vi "固定站CODMn测量流程.vi"(11 "控制命令":T1(ring)) -> ()   [LabVIEW 2016, in "斯坦道CODMn.lvlib"]
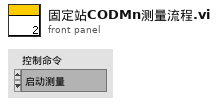
[diagram p1: front panel]
types:
  T1 = enum16{"启动测量", "标样核查", "零点核查", "跨度核查", "空白测试", "平行样测试", "加标回收", "空白校准", "标样校准", "初始化（清洗）", "停止测试", "仪器重启", "校时", "模式设置", "测量间隔设置"}
  T2 = cluster{"仪器":enum16{"", "氨氮", "总磷", "总氮", "CODMn", "CODCr"}, "启动命令":enum16{"启动水样流程", "启动加标流程", "排液", "停止", "柱塞泵启动"}}
  T3 = cluster{"时间标识":timestamp, "参数":string, "日志信息":string, "流程参数":string}
  T4 = cluster{"测量模式":enum16{"水样测量", "标样核查", "零点核查", "跨度核查", "空白测试", "加标回收", "平行样", "校零", "校标"}}
  T5 = cluster{"时间标识":timestamp, "设备":string, "日志信息":string, "流程参数":string}
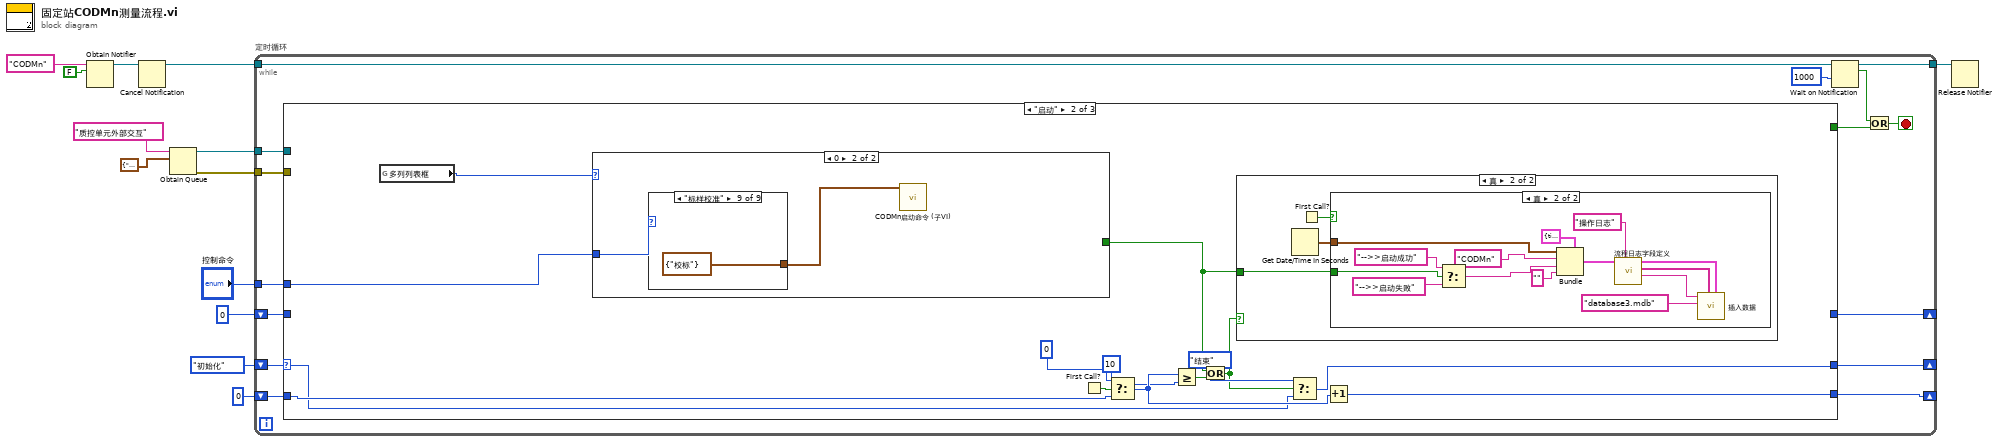
[diagram p0: block diagram]
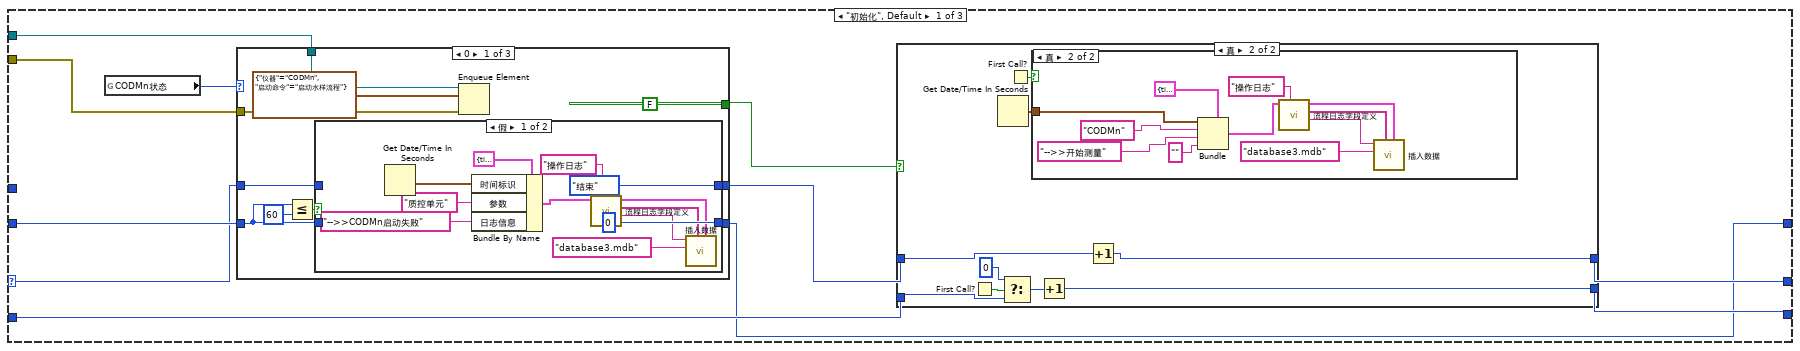
[diagram p2: hidden frame]
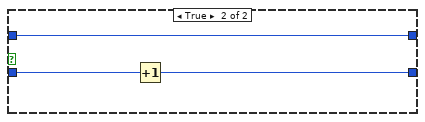
[diagram p5: hidden frame]
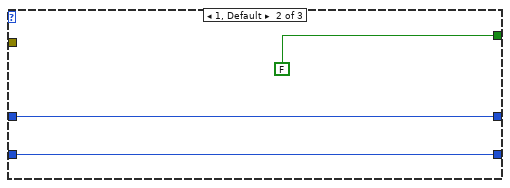
[diagram p6: hidden frame]
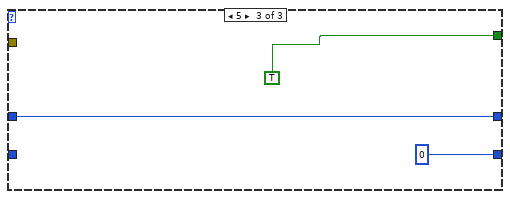
[diagram p7: hidden frame]
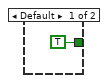
[diagram p10: hidden frame]
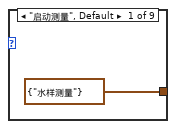
[diagram p11: hidden frame]
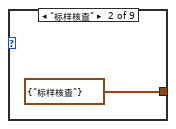
[diagram p12: hidden frame]
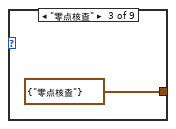
[diagram p13: hidden frame]
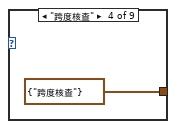
[diagram p14: hidden frame]
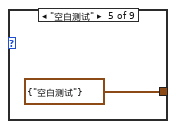
[diagram p15: hidden frame]
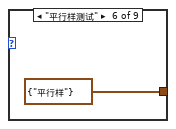
[diagram p16: hidden frame]
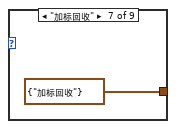
[diagram p17: hidden frame]
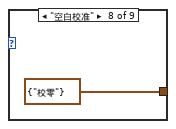
[diagram p18: hidden frame]
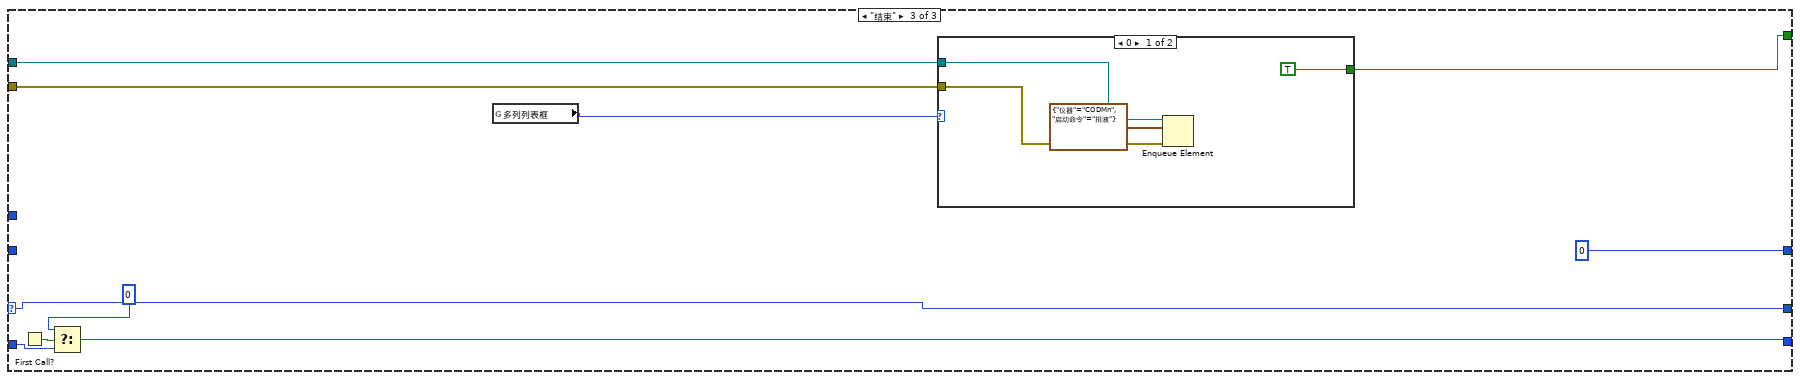
[diagram p19: hidden frame]
diagram:
  n1 = Obtain Notifier(name (unnamed)="CODMn" ("名称（未命名）"), notification data type=FALSE) -> (notifier out=w11:refnum<notifier>)  [unwired: 2 in, 2 out]
  n2 = Cancel Notification(0:w11) -> (8:w10:refnum<notifier>)  [unwired: 1 in, 2 out]
  n3 = Obtain Queue(name (unnamed)="质控单元外部交互" ("名称（未命名）"), element data type=T2 {"仪器"=enum."氨氮", "启动命令"=enum."启动水样流程"} ("元素")) -> (queue out=w3:refnum<queue>, error out=w2:errorcluster)  [unwired: 3 in, 1 out]
  n4 = while "定时循环" {
    tunnel: w10 -> [w28]
    tunnel: "控制命令" -> [w23]
    shift-right: [w22] -> _
    shift-left: enum16{"初始化", "启动", "结束"}."初始化" -> [w24]
    shift-right: [w20] -> _
    shift-left: 0 -> [w21]
    tunnel: [w18] -> w7
    tunnel: w3 -> [w17]
    tunnel: w2 -> [w16]
    shift-right: [w14] -> _
    shift-left: 0 -> [w15]
    stop <- w25 stop-if-true
    n5 = case shown="\"启动\"" w24 {
      selector: w24 -> [w31 w98 w145]
      tunnel: w23 -> [_ w106 _]
      tunnel: [w39 w99 w145] -> w22
      tunnel: w21 -> [w38 w103 w142]
      tunnel: [w37 w102 w141] -> w20
      tunnel: [_ _ w138] -> w19
      tunnel: w17 -> [w35 _ w140]
      tunnel: w16 -> [w34 _ w139]
      tunnel: w15 -> [w33 _ _]
      tunnel: [w32 _ 0] -> w14
      frame "初始化", Default {
        n6 = global read "CODMN外部API.vi" "CODMn状态"() -> (w29:u16)
        n7 = case shown="0" w29 {
          tunnel: [FALSE ("s") FALSE ("s") TRUE ("s")] -> w36
          tunnel: w35 -> [w70 _ _]
          tunnel: w34 -> [w69 _ _]
          tunnel: w33 -> [w67 w87 _]
          tunnel: [w64 w87 0] -> w32
          tunnel: w31 -> [w63 w88 w91]
          tunnel: [w62 w88 w91] -> w30
          frame 0 {
            n8 = Less Or Equal?(x=w67, y=60) -> (x <= y?=w65:bool)
            n9 = case shown="假" w65 {
              tunnel: w67 -> [_ w86]
              tunnel: [0 w85] -> w64
              tunnel: w63 -> [_ w84]
              tunnel: [enum16{"初始化", "启动", "结束"}."结束" w84] -> w62
              frame False {
                n10 = Get Date/Time In Seconds() -> (seconds since 1Jan1904=w79:timestamp)
                n11 = Bundle By Name(cluster=T3 {"时间标识"=timestamp(0 s since 1904-01-01), "参数"="", "日志信息"="", "流程参数"=""} ("data in"), "时间标识"=w79, "参数"="质控单元" ("设备"), "日志信息"="-->>CODMn启动失败") -> (w73:T3)
                n12 = call "流程日志字段定义.vi"("table输入"="操作日志", "data in"=w73) -> ("table输出"=w76:string, "columns"=w77:string[], "data out"=w78:T5)  [unwired: 7 in]
                n13 = call "插入数据.vi"("data"=w78, "columns"=w77, "database"="database3.mdb", "table"=w76) -> ()  [unwired: 7 in, 1 out]
              }
              frame True {
                n14 = Increment(x=w86) -> (x+1=w85:i32)
              }
            }
            n15 = Enqueue Element(queue=w70, element=T2 {"仪器"=enum."CODMn", "启动命令"=enum."启动水样流程"} ("元素"), error in (no error)=w69) -> ()  [unwired: 1 in, 3 out]
          }
          frame 1, Default {
          }
          frame 5 {
          }
        }
        n16 = case shown="真" w36 {
          tunnel: w30 -> [w41 w48]
          tunnel: [w41 w47] -> w39
          tunnel: w38 -> [w40 w45]
          tunnel: [w40 w42] -> w37
          frame False {
          }
          frame True {
            n17 = First Call?() -> (First Call?: T/F=w46:bool)
            n18 = Get Date/Time In Seconds() -> (seconds since 1Jan1904=w50:timestamp)
            n19 = Select(t=0, s=w46, f=w45) -> (s? t:f=w43:i32)
            n20 = First Call?() -> (First Call?: T/F=w49:bool)
            n21 = case shown="真" w49 {
              tunnel: w50 -> [_ w58]
              frame False {
              }
              frame True {
                n22 = Bundle(cluster=T3 {"时间标识"=timestamp(0 s since 1904-01-01), "参数"="", "日志信息"="", "流程参数"=""} ("data in"), "时间标识"=w58, "参数"="CODMn" ("设备"), "日志信息"="-->>开始测量", "流程参数"="" ("table输入")) -> (w51:T3)
                n23 = call "流程日志字段定义.vi"("table输入"="操作日志", "data in"=w51) -> ("table输出"=w54:string, "columns"=w53:string[], "data out"=w52:T5)  [unwired: 7 in]
                n24 = call "插入数据.vi"("data"=w52, "columns"=w53, "database"="database3.mdb", "table"=w54) -> ()  [unwired: 7 in, 1 out]
              }
            }
            n25 = Increment(x=w43) -> (x+1=w42:i32)
            n26 = Increment(x=w48) -> (x+1=w47:enum16{"初始化", "启动", "结束"})
          }
        }
      }
      frame "启动" {
        n27 = global read "运行时序全局变量.vi" "多列列表框"() -> (w93:i32)
        n28 = case shown="0" w93 {
          tunnel: w106 -> [_ w126]
          tunnel: [TRUE _] -> w94
          frame Default {
          }
          frame 0 {
            n29 = case shown="\"标样校准\"" w126 {
              tunnel: [T4 {"测量模式"=enum."水样测量"} ("启动测量模式") T4 {"测量模式"=enum."标样核查"} ("启动测量模式") T4 {"测量模式"=enum."零点核查"} ("启动测量模式") T4 {"测量模式"=enum."跨度核查"} ("启动测量模式") T4 {"测量模式"=enum."空白测试"} ("启动测量模式") T4 {"测量模式"=enum."平行样"} ("启动测量模式") T4 {"测量模式"=enum."加标回收"} ("启动测量模式") T4 {"测量模式"=enum."校零"} ("启动测量模式") T4 {"测量模式"=enum."校标"} ("启动测量模式")] -> w125
              frame "启动测量", Default {
              }
              frame "标样核查" {
              }
              frame "零点核查" {
              }
              frame "跨度核查" {
              }
              frame "空白测试" {
              }
              frame "平行样测试" {
              }
              frame "加标回收" {
              }
              frame "空白校准" {
              }
              frame "标样校准" {
              }
            }
            n30 = call "CODMn启动命令 (子VI).vi"("启动测量模式"=w125) -> ()  [unwired: 11 in]
          }
        }
        n31 = First Call?() -> (First Call?: T/F=w105:bool)
        n32 = Select(t=0, s=w105, f=w103) -> (s? t:f=w101:i32)
        n33 = Greater Or Equal?(x=w101, y=10) -> (x >= y?=w97:bool)
        n34 = Or(x=w94, y=w97) -> (x .or. y?=w95:bool)
        n35 = case shown="真" w95 {
          tunnel: w94 -> [_ w107]
          frame False {
          }
          frame True {
            n36 = Get Date/Time In Seconds() -> (seconds since 1Jan1904=w108:timestamp)
            n37 = First Call?() -> (First Call?: T/F=w109:bool)
            n38 = case shown="真" w109 {
              tunnel: w108 -> [_ w112]
              tunnel: w107 -> [_ w123]
              frame False {
              }
              frame True {
                n39 = Select(t="-->>启动成功" ("日志信息"), s=w123, f="-->>启动失败" ("日志信息")) -> (s? t:f=w110:string)
                n40 = Bundle(cluster=T3 {"时间标识"=timestamp(0 s since 1904-01-01), "参数"="", "日志信息"="", "流程参数"=""} ("data in"), "时间标识"=w112, "参数"="CODMn" ("设备"), "日志信息"=w110, "流程参数"="" ("table输入")) -> (w118:T3)
                n41 = call "流程日志字段定义.vi"("table输入"="操作日志", "data in"=w118) -> ("table输出"=w115:string, "columns"=w114:string[], "data out"=w113:T5)  [unwired: 7 in]
                n42 = call "插入数据.vi"("data"=w113, "columns"=w114, "database"="database3.mdb", "table"=w115) -> ()  [unwired: 7 in, 1 out]
              }
            }
          }
        }
        n43 = Select(t=enum16{"初始化", "启动", "结束"}."结束", s=w95, f=w98) -> (s? t:f=w99:enum16{"初始化", "启动", "结束"})
        n44 = Increment(x=w101) -> (x+1=w102:i32)
      }
      frame "结束" {
        n45 = First Call?() -> (First Call?: T/F=w144:bool)
        n46 = Select(t=0, s=w144, f=w142) -> (s? t:f=w141:i32)
        n47 = global read "运行时序全局变量.vi" "多列列表框"() -> (w136:i32)
        n48 = case shown="0" w136 {
          tunnel: w140 -> [w148 _]
          tunnel: w139 -> [w147 _]
          tunnel: [TRUE _] -> w138
          frame 0 {
            n49 = Enqueue Element(queue=w148, element=T2 {"仪器"=enum."CODMn", "启动命令"=enum."排液"} ("元素"), error in (no error)=w147) -> ()  [unwired: 1 in, 3 out]
          }
          frame 1, Default {
          }
        }
      }
    }
    n50 = Wait on Notification(notifier=w28, timeout in ms (-1)=1000 ("超时毫秒(-1)")) -> (notifier out=w18:refnum<notifier>, notification=w26:bool)  [unwired: 2 in, 2 out]
    n51 = Or(x=w26, y=w19) -> (x .or. y?=w25:bool)
  }
  n52 = Release Notifier(notifier=w7) -> ()  [unwired: 2 in, 3 out]
